vi "调试Auto.vi"   [LabVIEW 2018]
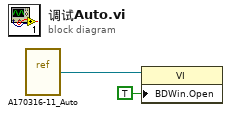
[diagram p0: block diagram]
diagram:
  n1 = vi-ref "A170316-11_Auto.vi"() -> (w2:refnum<vi>)
  n2 = property class="VI"(reference=w2, "BDWin.Open"=TRUE ("程序框图窗口:打开")) -> ()  [unwired: 1 in, 2 out]
